vi "Change Number's Digits.vi"(10 "precision (6)":i16, 11 "waveform":waveform(dbl)) -> (3 "output waveform":waveform(dbl))   [LabVIEW 2021]
doc: "减小数据的小数点后面的位数。\n2015-07-14 20:25:06\n蒋松\njiangsong@outlook.com"
panel:
  # "减小数据的小数点后面的位数。\n2015-07-14 20:25:06\n蒋松\njiangsong@outlook.com"
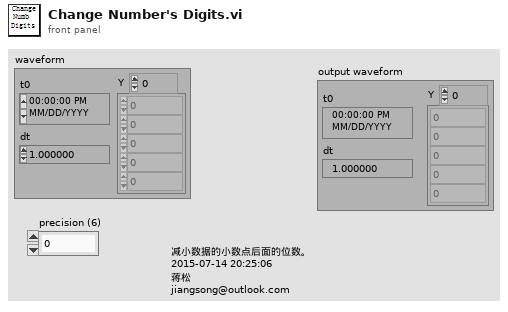
[diagram p1: front panel]
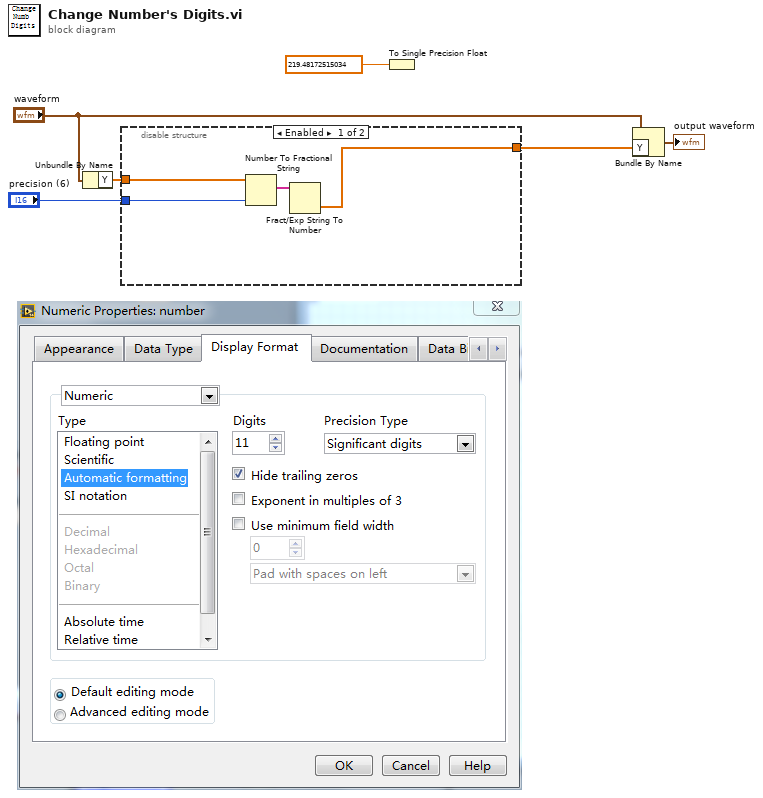
[diagram p0: block diagram]
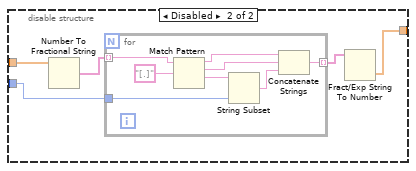
[diagram p2: hidden frame]
diagram:
  n1 = Unbundle By Name("waveform") -> ("Y"=w5:dbl[])
  n2 = disable-structure shown="Enabled" {
    disable-tunnel: w5 -> [w10 w15]
    disable-tunnel: "precision (6)" -> [w9 w13]
    disable-tunnel: [w8 w11] -> w2
    frame Enabled {
      n3 = Number To Fractional String(number=w10, precision (6)=w9) -> (F-format string=w7:string[])  [unwired: 2 in]
      n4 = Fract/Exp String To Number(string=w7) -> (number=w8:dbl[])  [unwired: 3 in, 1 out]
    }
    frame Disabled {
      n5 = Number To Fractional String(number=w15) -> (F-format string=w14:string[])  [unwired: 3 in]
      n6 = for {
        tunnel: w14 -> [w23] mode=indexing
        tunnel: w13 -> [w20]
        tunnel: [w16] -> w12 mode=indexing
        n7 = Match Pattern(string=w23, regular expression="[.]" ("search string")) -> (before substring=w19:string, match substring=w18:string, after substring=w21:string)  [unwired: 1 in, 1 out]
        n8 = String Subset(string=w21, length (rest)=w20) -> (substring=w17:string)  [unwired: 1 in]
        n9 = Concatenate Strings(w19, w18, w17) -> (w16:string)
      }
      n10 = Fract/Exp String To Number(string=w12) -> (number=w11:dbl[])  [unwired: 3 in, 1 out]
    }
  }
  n11 = To Single Precision Float(number=219.48172515034 ("Numeric")) -> ()  [unwired: 1 out]
  n12 = Bundle By Name(cluster="waveform", "Y"=w2) -> (→"output waveform":waveform(dbl))
